vi "SendFile2.vi"(4 "error in":errorcluster) -> (0 "error out":errorcluster, 1 "last ses time":timestamp)   [LabVIEW 2010]
uses:
  lib/Global 2.vi
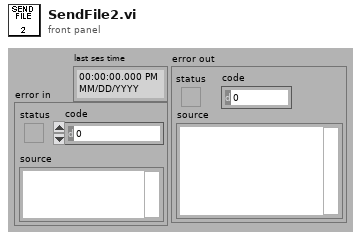
[diagram p1: front panel]
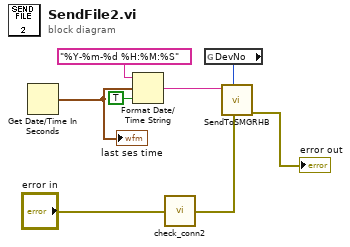
[diagram p0: block diagram]
diagram:
  n1 = Get Date/Time In Seconds() -> (seconds since 1Jan1904=w3:timestamp)
  "last ses time" <- w3
  n2 = Format Date/Time String(time format string (%c)="%Y-%m-%d %H:%M:%S", seconds (now)=w3, UTC format=TRUE) -> (date/time string=w6:string)
  n3 = call "check_conn2.vi"("error IO"="error in") -> ("error out"=w2:errorcluster)
  n4 = global read "Global 2.vi" "DevNo"() -> (w5:i32)
  n5 = call "SendToSMGRHB.vi"("error in"=w2, "meas_point"=w5, "date"=w6) -> ("error out"=→"error out":errorcluster)  [unwired: 6 in, 2 out]
